vi "Popup Image Window.vi"(11 "Event Passback":refnum<notifier>) -> ()   [LabVIEW 2020, in "AR Example.lvlib" / "UI.lvclass"]
uses:
  UI.lvclass
  Popup Image Window Events.ctl
  Popup Image Window Action.ctl
  g_ar_toolkit.image/Size (ARGB).vi
  g_ar_toolkit.image/Draw Image to Picture (ARGB).vi
  g_ar_toolkit.image/Size (ARGB).vi/69a1505b-b287-44ed-9ef9-f10ed7b260f4.vi
  g_ar_toolkit.image/Draw Image to Picture (ARGB).vi/8cd07b1b-062e-4fe4-9e87-2eb3dc89fe0e.vi
  g_ar_toolkit.common/Module Path.vi
  <vilib>/Utility/error.llb/Error Cluster From Error Code.vi
  UI.lvclass/UI.ctl
  g_ar_toolkit.image/g_ar_toolkit.image.lvlib
panel:
  out "Image":picture
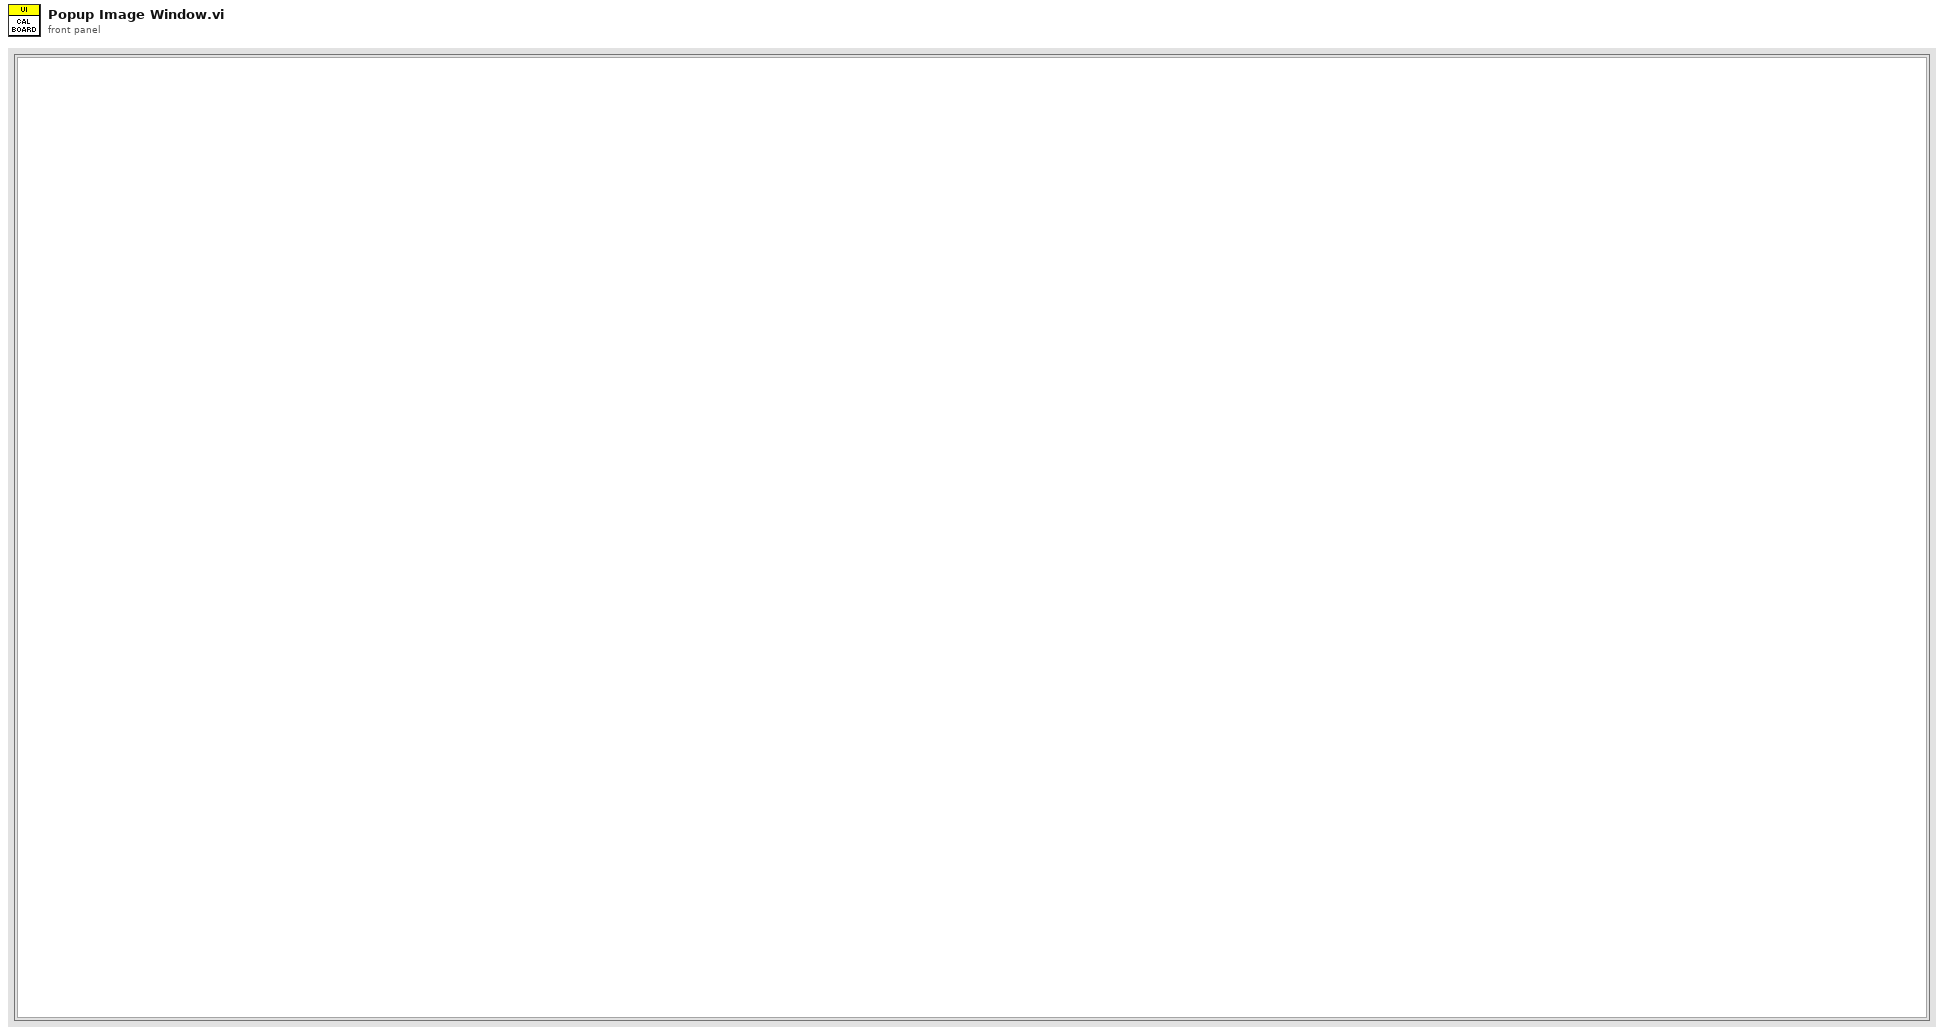
[diagram p1: front panel]
types:
  T1 = typedef "AR Example.lvlib/UI.lvclass/Popup Image Window Events.ctl" = cluster{"Update Image":refnum<user-event>, "Action":refnum<user-event>, "Update Window Name":refnum<user-event>}
  T2 = enum32{"Invalid", "Standard", "Closed", "Hidden", "Minimized", "Maximized"}
  T3 = typedef "g_ar_toolkit.common.lvlib/Image Size (Integer).ctl" = cluster{"Width":u16, "Height":u16}
  T4 = typedef "g_ar_toolkit.image.lvlib/ARGB Image.ctl" = refnum<data-value>
  T5 = typedef "g_ar_toolkit.image.lvlib/Image Draw Offset.ctl" = cluster{"Left":i16, "Top":i16}
  T6 = typedef "AR Example.lvlib/UI.lvclass/Popup Image Window Action.ctl" = enum16{"Show Panel", "Hide Panel", "Exit"}
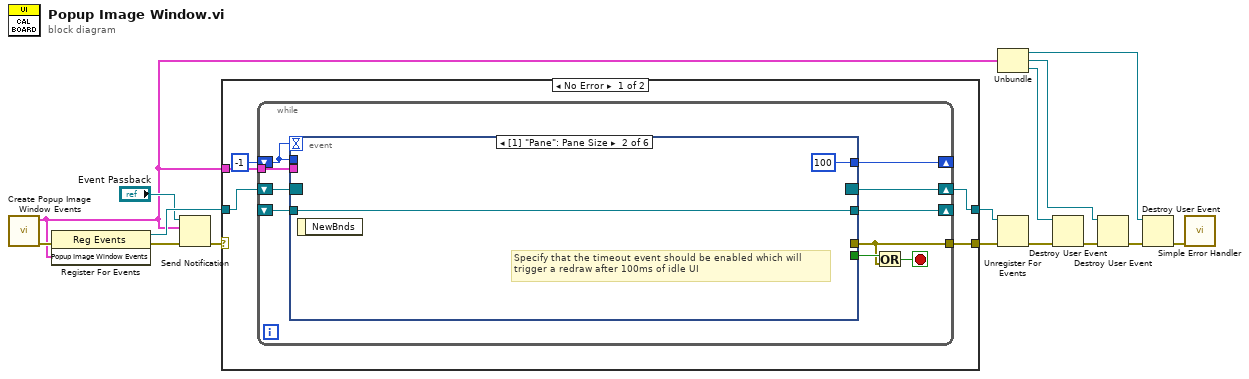
[diagram p0: block diagram]
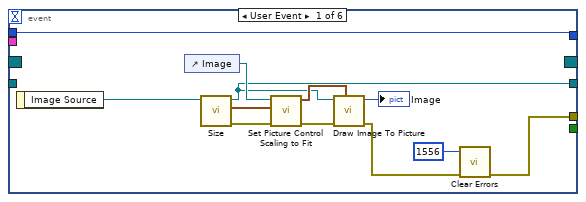
[diagram p2: hidden frame]
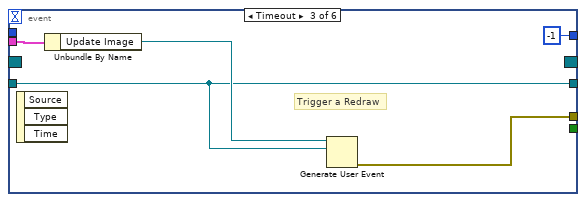
[diagram p3: hidden frame]
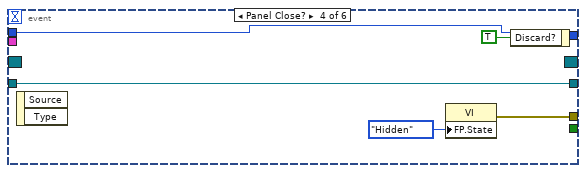
[diagram p4: hidden frame]
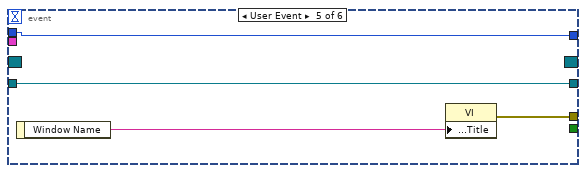
[diagram p5: hidden frame]
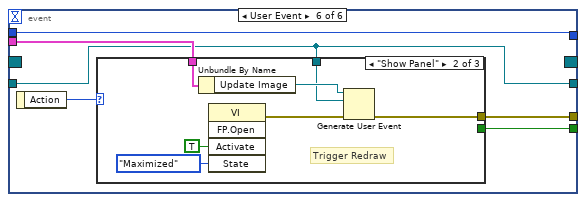
[diagram p6: hidden frame]
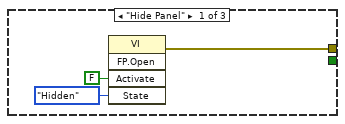
[diagram p7: hidden frame]
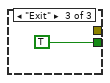
[diagram p8: hidden frame]
diagram:
  n1 = call "Create Popup Image Window Events.vi"() -> ("error out"=w14:errorcluster, "Popup Image Window Events"=w1:T1)  [unwired: 10 in]
  n2 = register-events(error in=w14, w1) -> (reference out=w15:refnum<event-registration>, error out=w13:errorcluster)  [unwired: 1 in]
  n3 = Send Notification(notification=w1, notifier="Event Passback", error in (no error)=w13) -> (error out=w11:errorcluster)  [unwired: 1 out]
  n4 = case shown="No Error" w11 {
    selector: w11 -> [_ w76]
    tunnel: w15 -> [w20 w77]
    tunnel: [w19 w77] -> w10
    tunnel: [w18 w76] -> w5
    tunnel: w1 -> [w17 _]
    frame No Error {
      n5 = while {
        shift-right: [w28] -> w19
        shift-left: w20 -> [w29]
        tunnel: [w26] -> w18
        shift-right: [w25] -> _
        shift-left: _ -> [w24]
        tunnel: w17 -> [w23]
        shift-right: [w22] -> _
        shift-left: -1 -> [w21]
        stop <- w30 stop-if-true
        n6 = event shown="[1] \"Pane\": Pane Size" {
          selector: w29 -> [_ _ _ _ _ _]
          dyn-events: [_ _ _ _ _ _] -> w28
          timeout: w21 -> [_ _ _ _ _ _]
          tunnel: [w33 _ w45 w52 w57 w64] -> w26
          tunnel: [_ _ _ _ _ w63] -> w27
          tunnel: [w34 w44 w46 w54 w56 w60] -> w25
          tunnel: w24 -> [_ w44 w46 w54 w56 w60]
          tunnel: w23 -> [_ _ w48 _ _ w61]
          tunnel: [w31 100 -1 w50 w55 w59] -> w22
          tunnel: w21 -> [w31 _ _ w50 w55 w59]
          event User Event {
            n7 = event-data() -> ("Image Source"=w40:refnum<data-value>)  [unwired: 1 in]
            n8 = control-ref of="Image"() -> (w39:refnum<vi>)
            n9 = call-poly "Size.vi"("ARGB Image"=w40) -> ("error out"=w38:errorcluster, "Image Size"=w36:T3, "ARGB Image (duplicate)"=w34:T4)  [unwired: 8 in]
            n10 = call "Set Picture Control Scaling to Fit.vi"("error in (no error)"=w38, "Image Size"=w36, "Picture in"=w39) -> ("error out"=w37:errorcluster, "Image Draw Offset"=w35:T5)  [unwired: 7 in]
            n11 = call-poly "Draw Image To Picture.vi"("Image Draw Offset (Default 0,0)"=w35, "error in (no error)"=w37, "ARGB Image Source"=w34) -> ("error out"=w42:errorcluster, "Picture"=→"Image":picture)  [unwired: 7 in]
            n12 = call <vilib>:"Clear Errors.vi"("error in (no error)"=w42, "specific error code to clear (0: all)"=1556) -> ("error out"=w33:errorcluster)  [unwired: 4 in, 1 out]
          }
          event Pane Size {
            # "Specify that the timeout event should be enabled which will\ntrigger a redraw after 100ms of idle UI"
            n13 = event-data() -> ()  [unwired: 1 in, 1 out]
          }
          event Timeout {
            # "Trigger a Redraw"
            n14 = event-data() -> ()  [unwired: 1 in, 3 out]
            n15 = Unbundle By Name(w48) -> ("Update Image"=w47:refnum<user-event>)
            n16 = Generate User Event(user event=w47, event data cluster=w46) -> (error out=w45:errorcluster)  [unwired: 2 in, 1 out]
          }
          event Panel Close? {
            n17 = event-data() -> ()  [unwired: 1 in, 2 out]
            n18 = property class="VI"("FP.State"=T2."Hidden" ("Front Panel Window:State")) -> (error out=w52:errorcluster)  [unwired: 2 in, 1 out]
            n19 = event-data("Discard?"=TRUE) -> ()  [unwired: 1 in, 1 out]
          }
          event User Event {
            n20 = event-data() -> ("Window Name"=w58:string)  [unwired: 1 in]
            n21 = property class="VI"("Front Panel.Title"=w58) -> (error out=w57:errorcluster)  [unwired: 2 in, 1 out]
          }
          event User Event {
            n22 = event-data() -> ("Action"=w62:T6)  [unwired: 1 in]
            n23 = case shown="\"Show Panel\"" w62 {
              tunnel: [w67 w69 _] -> w64
              tunnel: [_ _ TRUE] -> w63
              tunnel: w61 -> [_ w72 _]
              tunnel: w60 -> [_ w68 _]
              frame "Hide Panel" {
                n24 = invoke class="VI" method="FP.Open"("Activate"=FALSE ("Activate?"), "State"=T2."Hidden") -> (error out=w67:errorcluster)  [unwired: 3 in, 4 out]
              }
              frame "Show Panel" {
                # "Trigger Redraw"
                n25 = Unbundle By Name(w72) -> ("Update Image"=w71:refnum<user-event>)
                n26 = invoke class="VI" method="FP.Open"("Activate"=TRUE ("Activate?"), "State"=T2."Maximized" ("Front Panel Window:State")) -> (error out=w70:errorcluster)  [unwired: 3 in, 4 out]
                n27 = Generate User Event(user event=w71, event data cluster=w68, error in=w70) -> (error out=w69:errorcluster)  [unwired: 1 in, 1 out]
              }
              frame "Exit" {
              }
            }
          }
        }
        n28 = Or(x=w27, y=w26) -> (x .or. y?=w30:bool)
      }
    }
    frame Error {
    }
  }
  n29 = Unbundle(w1) -> ("Update Image"=w7:refnum<user-event>, "Action"=w9:refnum<user-event>, "Update Window Name"=w2:refnum<user-event>)
  n30 = Unregister For Events(event registration refnum=w10, error in=w5) -> (error out=w8:errorcluster)
  n31 = Destroy User Event(user event=w2, error in=w8) -> (error out=w3:errorcluster)
  n32 = Destroy User Event(user event=w9, error in=w3) -> (error out=w6:errorcluster)
  n33 = Destroy User Event(user event=w7, error in=w6) -> (error out=w4:errorcluster)
  n34 = call <vilib>:"Simple Error Handler.vi"("error in (no error)"=w4) -> ()  [unwired: 4 in, 5 out]
